vi "Read VKey.vi"(8 "error in (no error)":errorcluster, 11 "ControlKeyDownMsg in":refnum<class "VIKeyDownMsg.lvclass">) -> (0 "error out":errorcluster, 2 "VKey":T1, 3 "ControlKeyDownMsg out":refnum<class "VIKeyDownMsg.lvclass">)   [LabVIEW 2020, in "MVA Framework.lvlib" / "ActorEvents.lvlib" / "VIKeyDownMsg.lvclass"]
uses:
  VIKeyDownMsg.lvclass
  <vilib>/event_ctls.llb/eventvkey.ctl
  VIKeyDownMsg.lvclass/VIKeyDownMsg.ctl
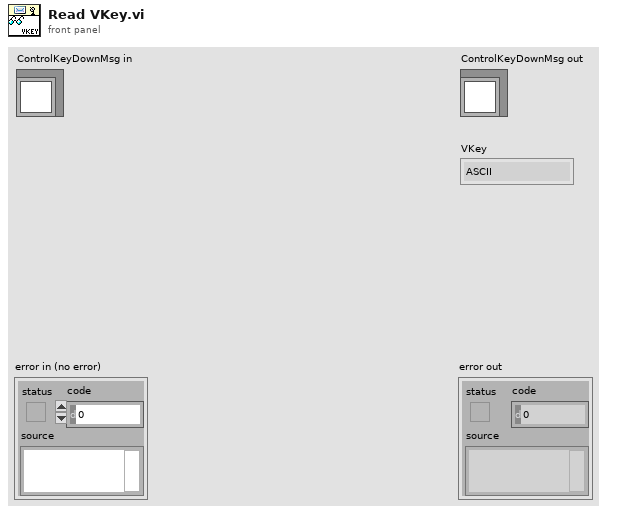
[diagram p1: front panel]
types:
  T1 = typedef "eventvkey.ctl" = enum16{"ASCII", "Enter", "Return", "Shift", "Ctrl", "Alt", "Cmd", "Opt", "Caps", "NumLock", "Clear", "Break", "Up", "Down", "Left", "Right", "Insert", "Delete", "Home", "End", "PageUp", "PageDown", "Escape", "Help", "Pause", "ScrollLock", "F1", "F2", "F3", "F4", "F5", "F6", "F7", "F8", "F9", "F10", "F11", "F12", "F13", "F14", "F15", "F16", "F17", "F18", "F19", "F20", "F21", "F22", "F23", "F24", "Play", "VolumeUp", "VolumeDown", "Mute", "Two Byte Char"}
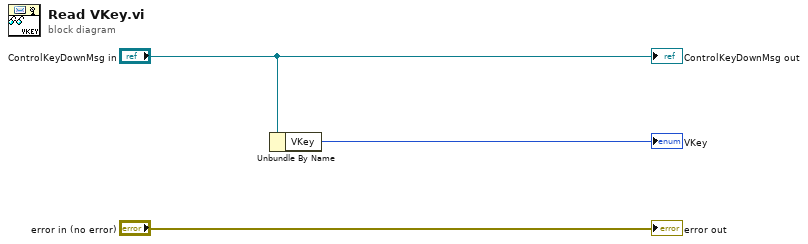
[diagram p0: block diagram]
diagram:
  n1 = Unbundle By Name("ControlKeyDownMsg in") -> ("VKey"=→"VKey":T1)
  "error out" <- "error in (no error)"
  "ControlKeyDownMsg out" <- "ControlKeyDownMsg in"
